vi "FTW-CodeGen-GetTypeInfoRemote.vi"(0 "Type Descriptor":i16[](array[numeric]) format="%04x", 5 "Type Data":string, 11 "error in":errorcluster) -> (4 "Data Type Color":u32(colorbox), 15 "error out":errorcluster)   [LabVIEW 2014]
panel:
  # "Inputs"
  # "Outputs"
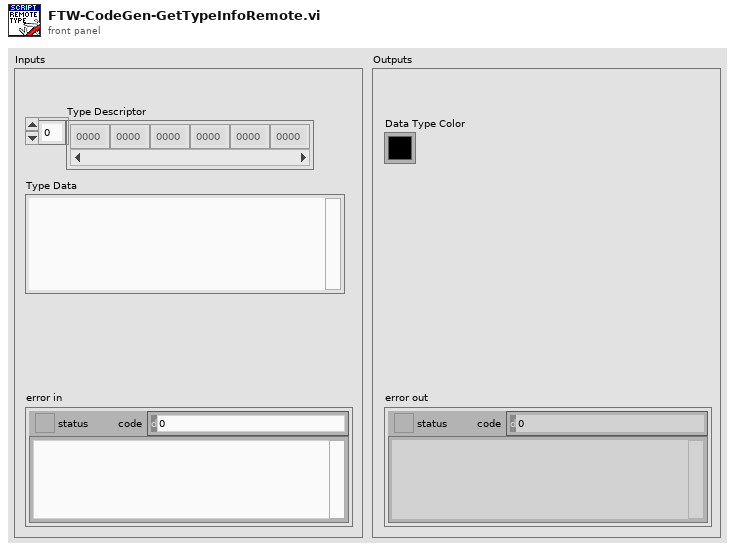
[diagram p1: front panel]
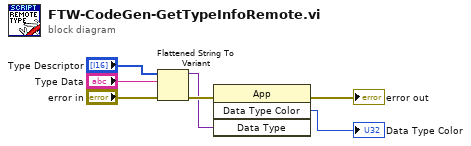
[diagram p0: block diagram]
diagram:
  n1 = Flattened String To Variant(4:"error in", 6:"Type Data", 7:"Type Descriptor") -> (0:w4:errorcluster, 3:w3:variant)
  n2 = invoke class="App" method="Data Type Color"(error in=w4, "Data Type"=w3) -> (error out=→"error out":errorcluster, "Data Type Color"=→"Data Type Color":u32)  [unwired: 2 in, 2 out]
